vi "Main.vi"() -> ()   [LabVIEW 2014]
uses:
  View/GraphSetting/TypeDef/WaveData.ctl
  Library/Event/Write User Event (Normal).vi
  View/GraphSetting/Dialog/Dialog GraphSetting (Chart).vi
  View/GraphSetting/Dialog/Dialog GraphSetting (Wave).vi
  <vilib>/measure/maspectr.llb/FFT Power Spectrum and PSD for 1 Chan.vi
  <vilib>/measure/NI_MABase.lvlib
  <vilib>/measure/NI_MAPro.lvlib
panel:
  out "波形チャート#1":dbl[][](graph)
  out "波形チャート #2":dbl[][](graph) caption="波形チャート#2"
  out "波形グラフ#1":cluster{"d0":dbl, "dt":dbl, "Y":dbl[]}[](graph)
  out "波形グラフ#2":cluster{"d0":dbl, "dt":dbl, "Y":dbl[]}[](graph)
  out "パワースペクトル#1":cluster{"f0":dbl, "df":dbl, "magnitude":dbl[]}[](graph)
  out "パワースペクトル#2":cluster{"f0":dbl, "df":dbl, "magnitude":dbl[]}[](graph)
  in  "環境設定ボタン":bool
  in  "終了ボタン":bool
  in  "再生ボタン":bool
  in  "記録ボタン":bool
  in  "設定ボタン":bool
  out "ボタン":u16
  in  "frequency":dbl=10.0 caption="周波数" format="%0.2p"
  in  "#s":dbl=1000.0
  in  "Fs":dbl=2000.0
  in  "ダミーデータ生成":bool
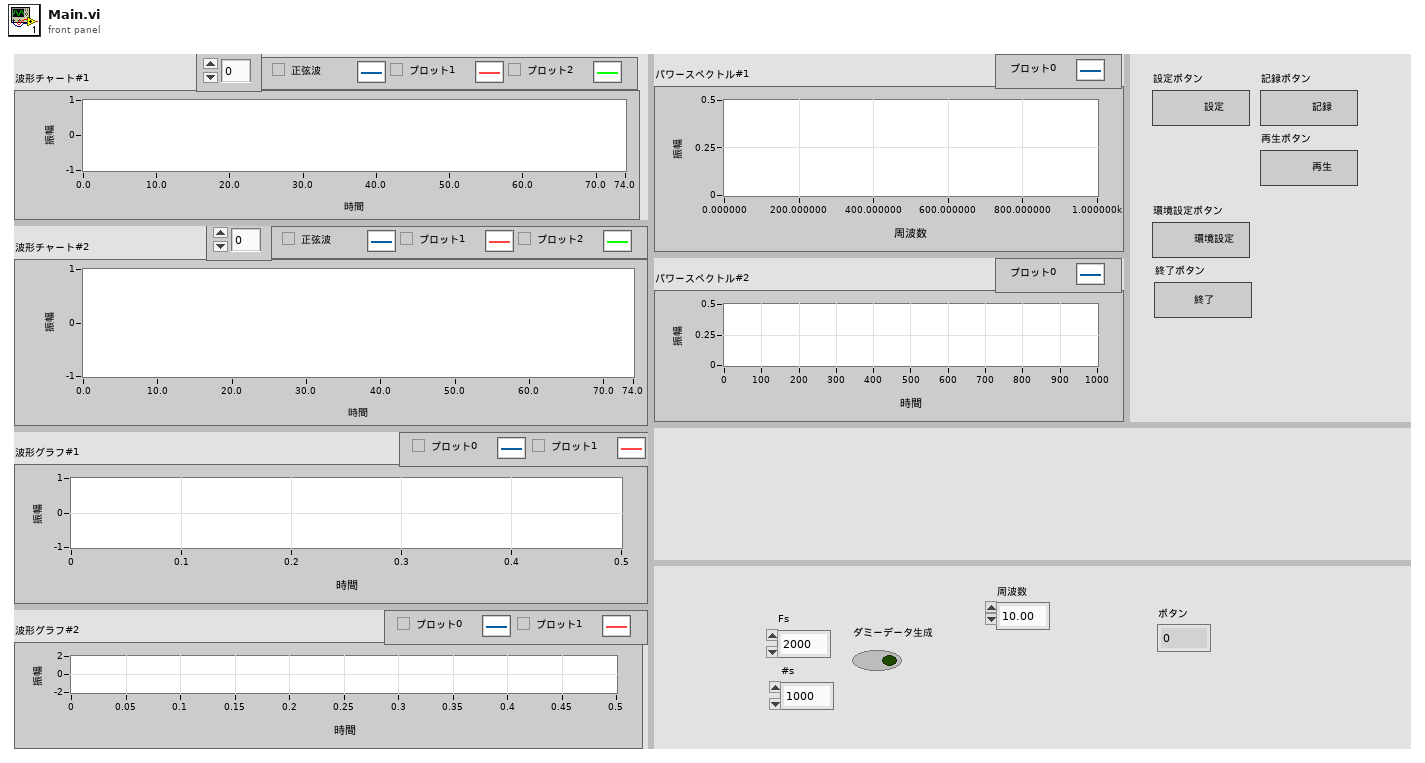
[diagram p1: front panel]
types:
  T1 = typedef "WaveData.ctl" = cluster{"d0":dbl, "dt":dbl, "Y":dbl[]}
  T2 = cluster{"queCMain":refnum<queue>, "queMMain":refnum<queue>, "queMWave#1":refnum<queue>, "queMWave#2":refnum<queue>}
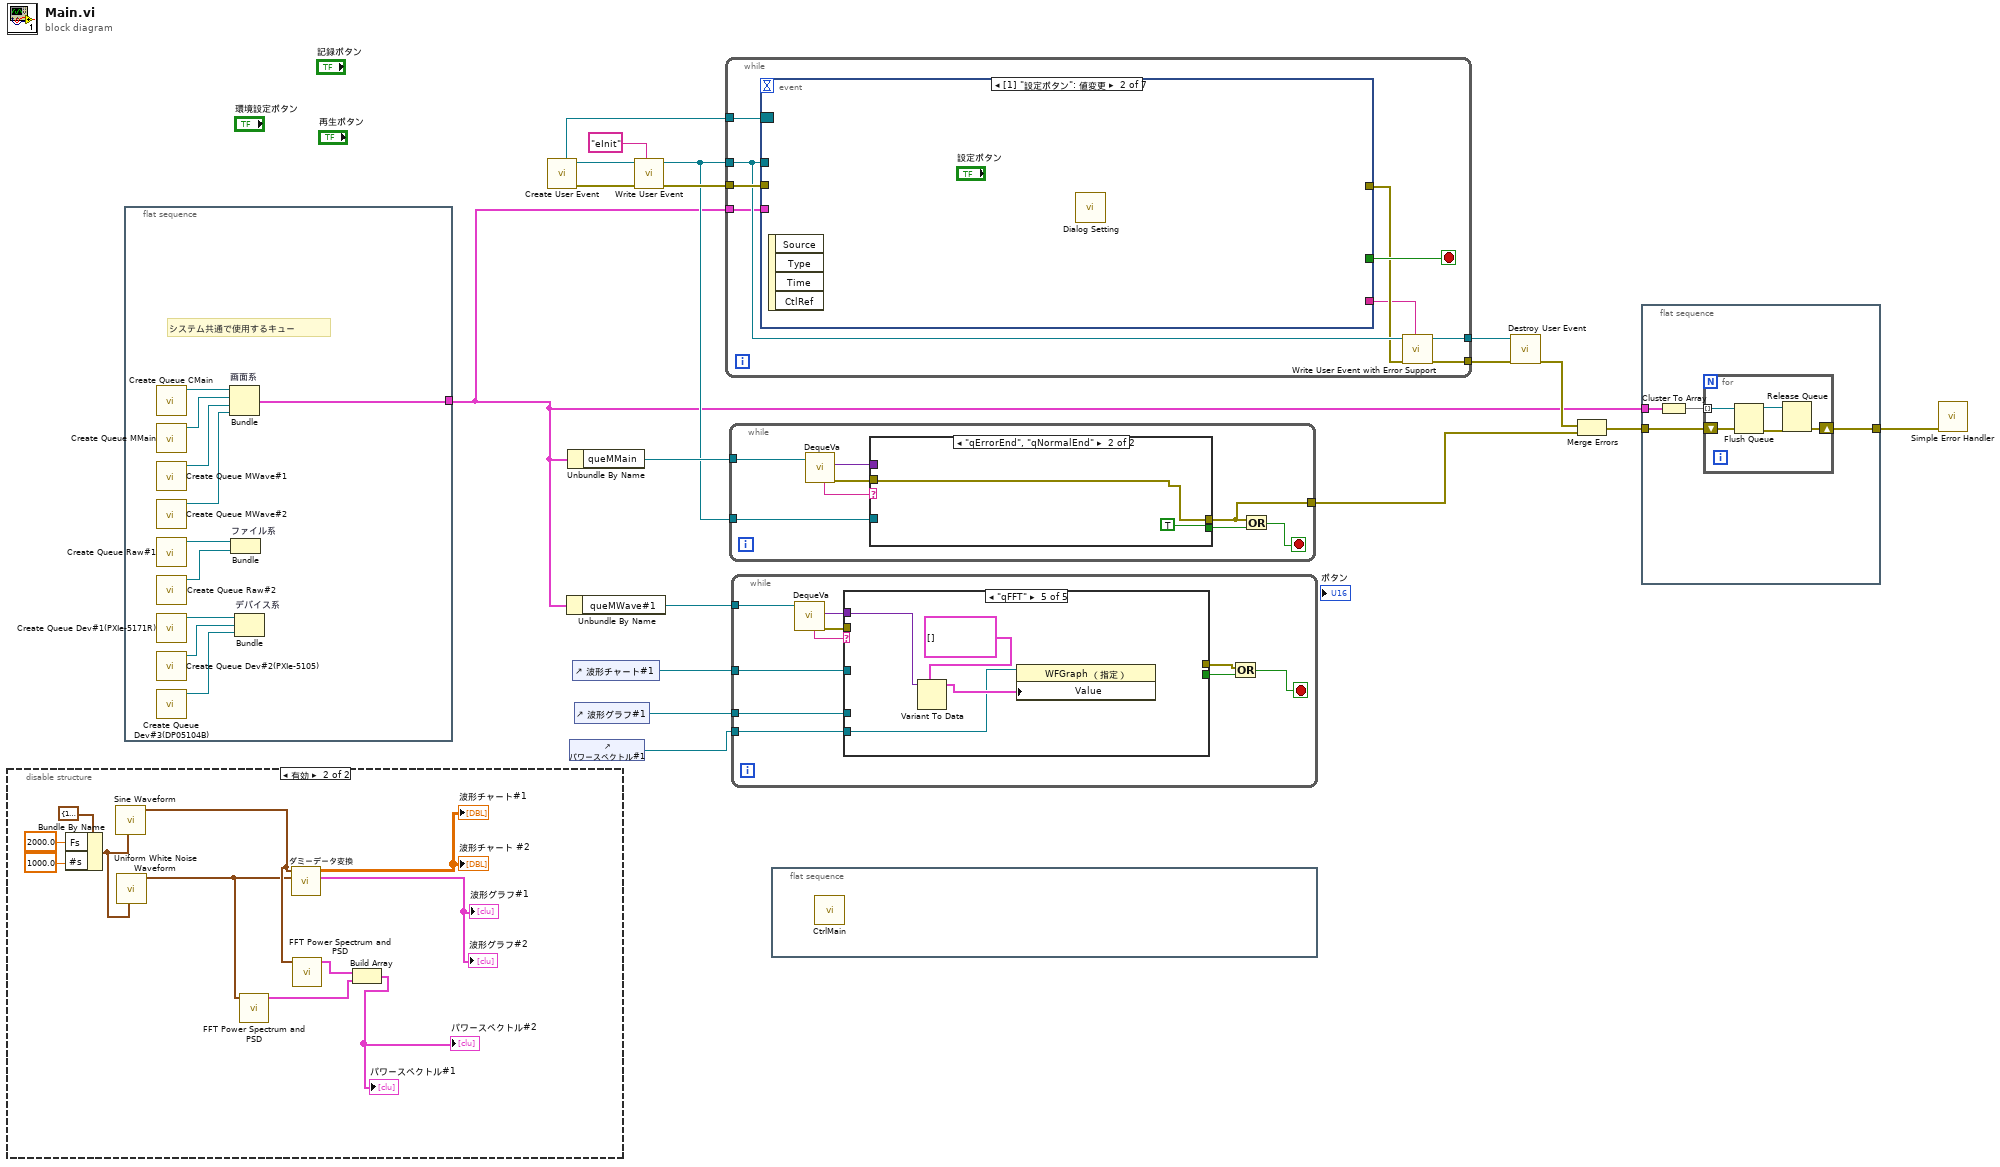
[diagram p0: block diagram]
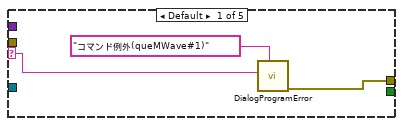
[diagram p3: hidden frame]
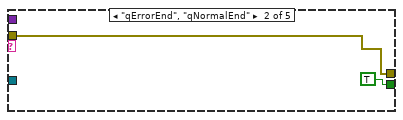
[diagram p4: hidden frame]
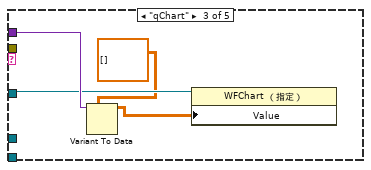
[diagram p5: hidden frame]
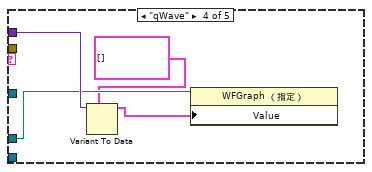
[diagram p6: hidden frame]
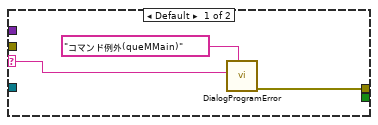
[diagram p7: hidden frame]
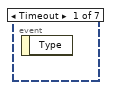
[diagram p8: hidden frame]
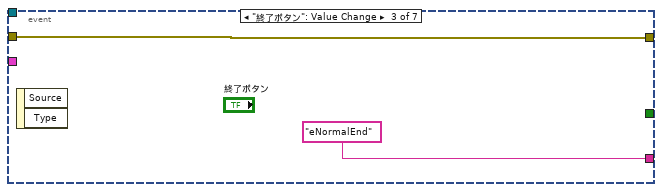
[diagram p9: hidden frame]
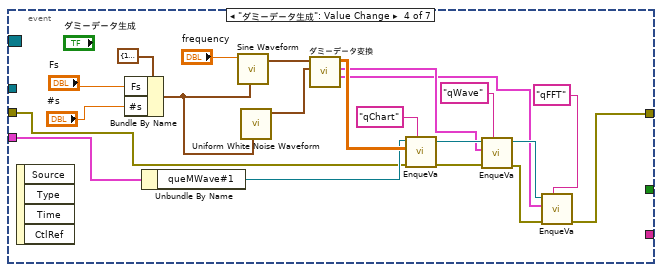
[diagram p10: hidden frame]
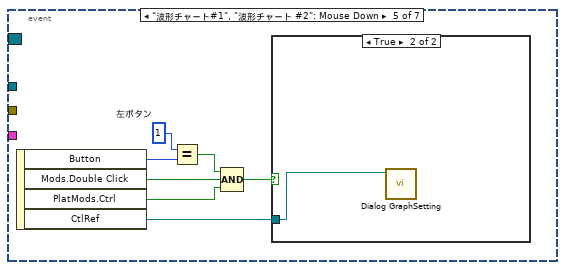
[diagram p11: hidden frame]
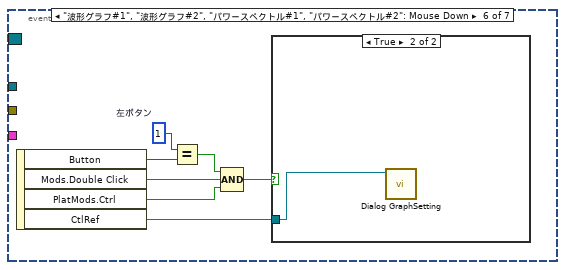
[diagram p13: hidden frame]
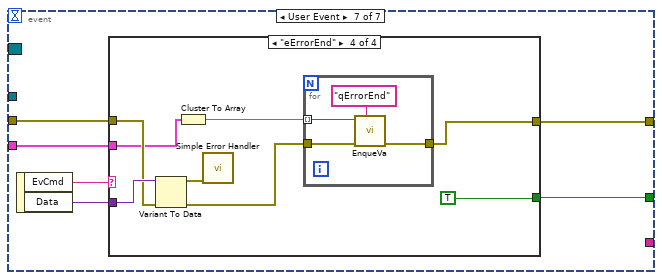
[diagram p15: hidden frame]
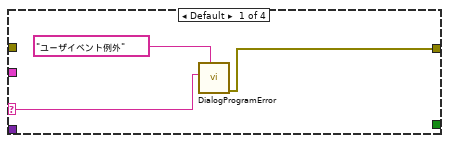
[diagram p16: hidden frame]
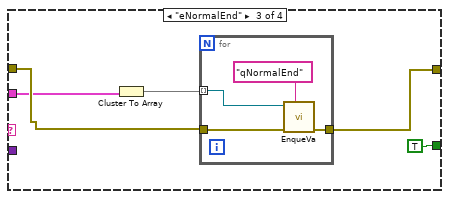
[diagram p18: hidden frame]
diagram:
  n1 = disable-structure shown="有効" {
    frame Disabled {
    }
    frame Enabled {
      n2 = Bundle By Name(cluster=cluster{"Fs":dbl, "#s":dbl} {"Fs"=1000.0, "#s"=1000.0} ("sampling info"), "Fs"=2000.0, "#s"=1000.0 ("Fs")) -> (w26:cluster{"Fs":dbl, "#s":dbl})
      n3 = call <vilib>:"Sine Waveform.vi"("sampling info"=w26) -> ("signal out"=w23:waveform(dbl))  [unwired: 9 in, 1 out]
      n4 = call <vilib>:"Uniform White Noise Waveform.vi"("sampling info"=w26) -> ("signal out"=w22:waveform(dbl))  [unwired: 9 in, 1 out]
      n5 = call-poly <vilib>:"FFT Power Spectrum and PSD.vi"("time signal"=w22) -> ("Power Spectrum / PSD"=w20:cluster{"f0":dbl, "df":dbl, "magnitude":dbl[]})  [unwired: 7 in, 3 out]
      n6 = call "ダミーデータ変換.vi"("signal out"=w22, "signal out 2"=w23) -> ("Wave[]"=→"波形グラフ#1" →"波形グラフ#2":T1[], "Chart[]"=→"波形チャート#1" →"波形チャート #2":dbl[][])  [unwired: 7 in, 1 out]
      n7 = call-poly <vilib>:"FFT Power Spectrum and PSD.vi"("time signal"=w23) -> ("Power Spectrum / PSD"=w21:cluster{"f0":dbl, "df":dbl, "magnitude":dbl[]})  [unwired: 7 in, 3 out]
      n8 = Build Array(w21, w20) -> (→"パワースペクトル#1" →"パワースペクトル#2":cluster{"f0":dbl, "df":dbl, "magnitude":dbl[]}[])
    }
  }
  n9 = flat-sequence {
    tunnel: [w30] -> w4
    frame #0 {
      # "システム共通で使用するキュー"
      n10 = call "Create Queue CMain.vi"() -> ("queCMain"=w39:refnum<queue>)  [unwired: 10 in, 1 out]
      n11 = call "Create Queue MMain.vi"() -> ("queMMain"=w38:refnum<queue>)  [unwired: 10 in, 1 out]
      n12 = call "Create Queue MWave#1.vi"() -> ("queMWave#1"=w37:refnum<queue>)  [unwired: 10 in, 1 out]
      n13 = call "Create Queue MWave#2.vi"() -> ("queMWave#2"=w36:refnum<queue>)  [unwired: 10 in, 1 out]
      n14 = call "Create Queue Raw#1.vi"() -> ("queRaw#1"=w35:refnum<queue>)  [unwired: 10 in, 1 out]
      n15 = call "Create Queue Raw#2.vi"() -> ("queRaw#2"=w34:refnum<queue>)  [unwired: 10 in, 1 out]
      n16 = call "Create Queue Dev#1(PXIe-5171R).vi"() -> ("queDev#1"=w33:refnum<queue>)  [unwired: 10 in, 1 out]
      n17 = call "Create Queue Dev#2(PXIe-5105).vi"() -> ("queDev#2"=w32:refnum<queue>)  [unwired: 10 in, 1 out]
      n18 = call "Create Queue Dev#3(DP05104B).vi"() -> ("queDev#3"=w31:refnum<queue>)  [unwired: 10 in, 1 out]
      n19 = Bundle "画面系"("queCMain"=w39, "queMMain"=w38, "queMWave#1"=w37, "queMWave#2"=w36) -> (w30:T2)  [unwired: 1 in]
      n20 = Bundle "ファイル系"("queRaw#1"=w35, "queRaw#2"=w34) -> ()  [unwired: 1 in, 1 out]
      n21 = Bundle "デバイス系"("queDev#1"=w33, "queDev#2"=w32, "queDev#3"=w31) -> ()  [unwired: 1 in, 1 out]
    }
  }
  n22 = call "Create User Event.vi"() -> ("error out"=w18:errorcluster, "User Event"=w17:refnum<user-event>, "Event Registration Refnum"=w15:refnum<event-registration>)  [unwired: 9 in]
  n23 = Unbundle By Name(w4) -> ("queMWave#1"=w5:refnum<queue>)
  n24 = Unbundle By Name(w4) -> ("queMMain"=w8:refnum<queue>)
  n25 = control-ref of="パワースペクトル#1"() -> (w1:refnum<vi>)
  n26 = control-ref of="波形チャート#1"() -> (w3:refnum<vi>)
  n27 = control-ref of="波形グラフ#1"() -> (w2:refnum<vi>)
  n28 = call-poly "Write User Event.vi"("EvCmd"="eInit", "エラー入力（エラーなし）"=w18, "ユーザイベント入力"=w17) -> ("エラー出力"=w14:errorcluster, "ユーザイベント出力"=w7:refnum<user-event>)  [unwired: 7 in]
  n29 = while {
    tunnel: w7 -> [w46]
    tunnel: w15 -> [w48]
    tunnel: w14 -> [w47]
    tunnel: [w42] -> w13
    tunnel: [w41] -> w12
    tunnel: w4 -> [w40]
    stop <- w45 stop-if-true
    n30 = event shown="[1] \"設定ボタン\": 値変更" {
      selector: w48 -> [_ _ _ _ _ _ _]
      dyn-events: _ -> [_ _ _ _ _ _ _]
      timeout: _ -> [_ _ _ _ _ _ _]
      tunnel: w46 -> [_ _ _ _ _ _ _]
      tunnel: w47 -> [_ _ w50 w58 _ _ w90]
      tunnel: [_ _ w50 w52 _ _ w88] -> w44
      tunnel: [_ _ _ _ _ _ w91] -> w45
      tunnel: [_ _ "eNormalEnd" ("EvCmd") _ _ _ _] -> w43
      tunnel: w40 -> [_ _ _ w66 _ _ w89]
      event Timeout {
        n31 = event-data() -> ()  [unwired: 1 in, 1 out]
      }
      event "設定ボタン": Value Change {
        n32 = event-data() -> ()  [unwired: 1 in, 4 out]
        n33 = call "Dialog Setting.vi"() -> ()  [unwired: 11 in, 1 out]
      }
      event "終了ボタン": Value Change {
        n34 = event-data() -> ()  [unwired: 1 in, 2 out]
      }
      event "ダミーデータ生成": Value Change {
        n35 = event-data() -> ()  [unwired: 1 in, 4 out]
        n36 = Bundle By Name(cluster=cluster{"Fs":dbl, "#s":dbl} {"Fs"=1000.0, "#s"=1000.0} ("sampling info"), "Fs"="Fs", "#s"="#s") -> (w70:cluster{"Fs":dbl, "#s":dbl})
        n37 = Unbundle By Name(w66) -> ("queMWave#1"=w63:refnum<queue>)
        n38 = call <vilib>:"Sine Waveform.vi"("sampling info"=w70, "frequency"="frequency") -> ("signal out"=w57:waveform(dbl))  [unwired: 8 in, 1 out]
        n39 = call <vilib>:"Uniform White Noise Waveform.vi"("sampling info"=w70) -> ("signal out"=w56:waveform(dbl))  [unwired: 9 in, 1 out]
        n40 = call "ダミーデータ変換.vi"("signal out"=w56, "signal out 2"=w57) -> ("パワースペクトル"=w51:cluster{"f0":dbl, "df":dbl, "magnitude":dbl[]}[], "Wave[]"=w60:T1[], "Chart[]"=w64:dbl[][])  [unwired: 7 in]
        n41 = call "EnqueVa.vi"("コマンド"="qChart", "エラー入力（エラーなし）"=w58, "バリアント"=w64, "queVariant"=w63) -> ("エラー出力"=w59:errorcluster, "queVariant(copy)"=w61:refnum<queue>)  [unwired: 5 in, 1 out]
        n42 = call "EnqueVa.vi"("コマンド"="qWave", "エラー入力（エラーなし）"=w59, "バリアント"=w60, "queVariant"=w61) -> ("エラー出力"=w53:errorcluster, "queVariant(copy)"=w54:refnum<queue>)  [unwired: 5 in, 1 out]
        n43 = call "EnqueVa.vi"("コマンド"="qFFT", "エラー入力（エラーなし）"=w53, "バリアント"=w51, "queVariant"=w54) -> ("エラー出力"=w52:errorcluster)  [unwired: 5 in, 2 out]
      }
      event "波形チャート#1", "波形チャート #2": Mouse Down {
        w77 = u16 1  # 左ボタン
        n44 = event-data() -> ("Button"=w78:u16, "Mods.Double Click"=w75:bool, "PlatMods.Ctrl"=w74:bool, "CtlRef"=w72:refnum<vi>)  [unwired: 1 in]
        n45 = Equal?(x=w77, y=w78) -> (x = y?=w76:bool)
        n46 = Compound Arithmetic op=AND ("複合演算")(w76, w75, w74) -> (w73:bool)
        n47 = case shown="TRUE" w73 {
          tunnel: w72 -> [_ w79]
          frame False {
          }
          frame True {
            n48 = call-poly "Dialog GraphSetting.vi"("波形チャートref(in)"=w79) -> ()  [unwired: 11 in]
          }
        }
      }
      event "波形グラフ#1", "波形グラフ#2", "パワースペクトル#1", "パワースペクトル#2": Mouse Down {
        w85 = u16 1  # 左ボタン
        n49 = event-data() -> ("Button"=w86:u16, "Mods.Double Click"=w83:bool, "PlatMods.Ctrl"=w82:bool, "CtlRef"=w80:refnum<vi>)  [unwired: 1 in]
        n50 = Equal?(x=w85, y=w86) -> (x = y?=w84:bool)
        n51 = Compound Arithmetic op=AND ("複合演算")(w84, w83, w82) -> (w81:bool)
        n52 = case shown="TRUE" w81 {
          tunnel: w80 -> [_ w87]
          frame False {
          }
          frame True {
            n53 = call-poly "Dialog GraphSetting.vi"("波形グラフref(in)"=w87) -> ()  [unwired: 11 in]
          }
        }
      }
      event User Event {
        n54 = event-data() -> ("EvCmd"=w93:string, "Data"=w92:variant)  [unwired: 1 in]
        n55 = case shown="\"eErrorEnd\"" w93 {
          selector: w93 -> [w95 _ _ _]
          tunnel: w92 -> [_ _ _ w112]
          tunnel: [_ _ TRUE TRUE] -> w91
          tunnel: w90 -> [_ _ w100 w110]
          tunnel: w89 -> [_ _ w98 w107]
          tunnel: [w94 _ w99 w109] -> w88
          frame Default {
            n56 = call "DialogProgramError.vi"("エラー内容"="ユーザイベント例外" ("エラー詳細"), "エラー詳細"=w95) -> ("error out"=w94:errorcluster)  [unwired: 9 in]
          }
          frame "eInit" {
          }
          frame "eNormalEnd" {
            n57 = Cluster To Array(cluster=w98) -> (array=w97:refnum<queue>[])
            n58 = for {
              tunnel: w100 -> [w104]
              tunnel: [w103] -> w99
              tunnel: w97 -> [w102] mode=indexing
              n59 = call "EnqueVa.vi"("コマンド"="qNormalEnd", "エラー入力（エラーなし）"=w104, "queVariant"=w102) -> ("エラー出力"=w103:errorcluster)  [unwired: 6 in, 2 out]
            }
          }
          frame "eErrorEnd" {
            n60 = Variant To Data(error in=w110, Variant=w112) -> (data=w111:errorcluster, error out=w108:errorcluster)  [unwired: 1 in]
            n61 = Cluster To Array(cluster=w107) -> (array=w106:refnum<queue>[])
            n62 = call <vilib>:"Simple Error Handler.vi"("error in (no error)"=w111) -> ()  [unwired: 4 in, 5 out]
            n63 = for {
              tunnel: w106 -> [w116] mode=indexing
              tunnel: [w115] -> w109
              tunnel: w108 -> [w114]
              n64 = call "EnqueVa.vi"("コマンド"="qErrorEnd", "エラー入力（エラーなし）"=w114, "queVariant"=w116) -> ("エラー出力"=w115:errorcluster)  [unwired: 6 in, 2 out]
            }
          }
        }
      }
    }
    n65 = call "Write User Event with Error Support.vi"("EvCmd"=w43, "エラー入力（エラーなし）"=w44, "ユーザイベント入力"=w46) -> ("エラー出力"=w41:errorcluster, "ユーザイベント出力"=w42:refnum<user-event>)  [unwired: 7 in]
  }
  n66 = while {
    tunnel: w8 -> [w125]
    tunnel: w7 -> [w119]
    tunnel: [w118] -> w6
    stop <- w120 stop-if-true
    n67 = call "DequeVa.vi"("queVariant"=w125) -> ("エラー出力"=w122:errorcluster, "バリアント"=w123:variant, "コマンド"=w124:string)  [unwired: 6 in, 2 out]
    n68 = case shown="\"qErrorEnd\", \"qNormalEnd\"" w124 {
      selector: w124 -> [w126 _]
      tunnel: w123 -> [_ _]
      tunnel: w122 -> [_ w129]
      tunnel: [_ TRUE] -> w121
      tunnel: [w128 w129] -> w118
      tunnel: w119 -> [_ _]
      frame Default {
        n69 = call "DialogProgramError.vi"("エラー内容"="コマンド例外(queMMain)" ("エラー詳細"), "エラー詳細"=w126) -> ("error out"=w128:errorcluster)  [unwired: 9 in]
      }
      frame "qErrorEnd", "qNormalEnd" {
      }
    }
    n70 = Or(x=w118, y=w121) -> (x .or. y?=w120:bool)
  }
  n71 = while {
    tunnel: w5 -> [w140]
    tunnel: w3 -> [w133]
    tunnel: w2 -> [w132]
    tunnel: w1 -> [w131]
    stop <- w137 stop-if-true
    n72 = call "DequeVa.vi"("queVariant"=w140) -> ("エラー出力"=w134:errorcluster, "バリアント"=w135:variant, "コマンド"=w139:string)  [unwired: 6 in, 2 out]
    n73 = case shown="\"qFFT\"" w139 {
      selector: w139 -> [w142 _ _ _ _]
      tunnel: [_ TRUE _ _ _] -> w138
      tunnel: [w141 w144 _ _ _] -> w136
      tunnel: w135 -> [_ _ w149 w153 w157]
      tunnel: w134 -> [_ w144 _ _ _]
      tunnel: w133 -> [_ _ w148 _ _]
      tunnel: w132 -> [_ _ _ w152 _]
      tunnel: w131 -> [_ _ _ _ w154]
      frame Default {
        n74 = call "DialogProgramError.vi"("エラー内容"="コマンド例外(queMWave#1)" ("エラー詳細"), "エラー詳細"=w142) -> ("error out"=w141:errorcluster)  [unwired: 9 in]
      }
      frame "qErrorEnd", "qNormalEnd" {
      }
      frame "qChart" {
        n75 = Variant To Data(type=dbl[][] [], Variant=w149) -> (data=w146:dbl[][])  [unwired: 1 in, 1 out]
        n76 = property class="WFChart （指定）"(reference=w148, "Value"=w146) -> ()  [unwired: 1 in, 2 out]
      }
      frame "qWave" {
        n77 = Variant To Data(type=T1[] [], Variant=w153) -> (data=w150:T1[])  [unwired: 1 in, 1 out]
        n78 = property class="WFGraph （指定）"(reference=w152, "Value"=w150) -> ()  [unwired: 1 in, 2 out]
      }
      frame "qFFT" {
        n79 = Variant To Data(type=T1[] [], Variant=w157) -> (data=w155:T1[])  [unwired: 1 in, 1 out]
        n80 = property class="WFGraph （指定）"(reference=w154, "Value"=w155) -> ()  [unwired: 1 in, 2 out]
      }
    }
    n81 = Or(x=w136, y=w138) -> (x .or. y?=w137:bool)
  }
  n82 = flat-sequence {
    frame #0 {
      n83 = call "CtrlMain.vi"() -> ()  [unwired: 12 in]
    }
  }
  n84 = call "Destroy User Event.vi"("error in (no error)"=w12, "User Event"=w13) -> ("error out"=w9:errorcluster)  [unwired: 9 in]
  n85 = Merge Errors(w9, w6) -> (w10:errorcluster)
  n86 = flat-sequence {
    tunnel: w4 -> [w161]
    tunnel: w10 -> [w159]
    tunnel: [w158] -> w11
    frame #0 {
      n87 = Cluster To Array(cluster=w161) -> (array=w160:refnum<queue>[])
      n88 = for {
        tunnel: w160 -> [w166] mode=indexing
        shift-right: [w163] -> w158
        shift-left: w159 -> [w162]
        n89 = Flush Queue(queue=w166, error in (no error)=w162) -> (queue out=w164:refnum<queue>, error out=w165:errorcluster)  [unwired: 1 out]
        n90 = Release Queue(queue=w164, error in (no error)=w165) -> (error out=w163:errorcluster)  [unwired: 1 in, 2 out]
      }
    }
  }
  n91 = call <vilib>:"Simple Error Handler.vi"("error in (no error)"=w11) -> ()  [unwired: 4 in, 5 out]
